vi "Mono Mirror.vi"(8 "error in (no error)":errorcluster, 11 "Mono In":refnum<class "Monochromator.lvclass">) -> (0 "error out":errorcluster, 2 "new Position":i32, 3 "Position":i32)   [LabVIEW 2020, in "Examples.lvlib"]
doc: "This example shows how to get and set the mirror position of the mono."
uses:
  Examples.lvlib
  Classes/Mono/Monochromator.lvclass
  0bd624ee-cc67-429d-86ba-aa8b37d700b1.vi
  01530acb-cdb4-4e7f-ad8c-3491b7af0b5d.vi
panel:
  in  "Stop":bool
  # "Connector Pane"
  # "Locals"
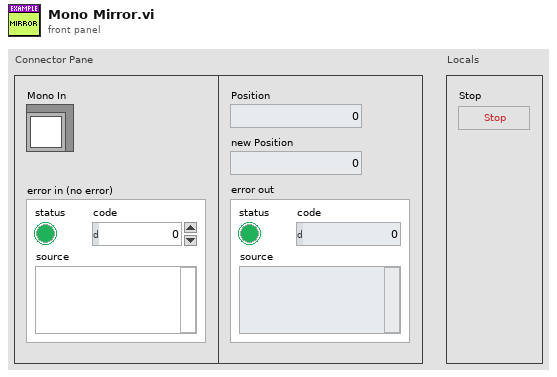
[diagram p1: front panel]
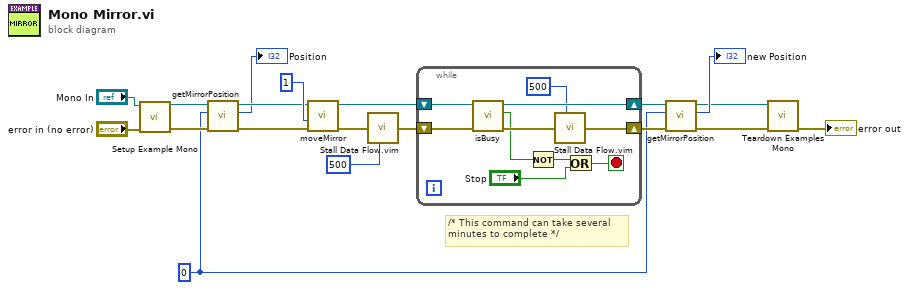
[diagram p0: block diagram]
diagram:
  w1 = 0 ("locationId")
  # "/* This command can take several \nminutes to complete */"
  n1 = call "Setup Example Mono.vi"("error in (no error)"="error in (no error)", "Mono In"="Mono In") -> ("error out"=w6:errorcluster, "Mono Out"=w4:refnum<class "Monochromator.lvclass">)  [unwired: 6 in, 2 out]
  n2 = call "getMirrorPosition.vi"("error in (no error)"=w6, "locationId"=w1, "Monochromator in"=w4) -> ("error out"=w5:errorcluster, "position"=→"Position":i32, "Monochromator out"=w3:refnum<class "Monochromator.lvclass">)  [unwired: 6 in]
  n3 = call "moveMirror.vi"("error in (no error)"=w5, "position"=1, "Monochromator in"=w3) -> ("error out"=w15:errorcluster, "Monochromator out"=w12:refnum<class "Monochromator.lvclass">)  [unwired: 5 in, 2 out]
  n4 = call "Stall Data Flow.vim"("value in"=w15, "milliseconds to wait"=u32 500) -> ("value out"=w14:errorcluster)  [unwired: 1 out]
  n5 = while {
    shift-right: [w25] -> w9
    shift-left: w14 -> [w27]
    shift-right: [w28] -> w10
    shift-left: w12 -> [w26]
    stop <- w22 stop-if-true
    n6 = call "isBusy.vi"("error in (no error)"=w27, "Monochromator in"=w26) -> ("error out"=w29:errorcluster, "mono is busy?"=w23:bool, "Monochromator out"=w28:refnum<class "Monochromator.lvclass">)  [unwired: 7 in]
    n7 = Not(x=w23) -> (.not. x?=w20:bool)
    n8 = call "Stall Data Flow.vim"("value in"=w29, "milliseconds to wait"=u32 500) -> ("value out"=w25:errorcluster)  [unwired: 1 out]
    n9 = Or(x=w20, y="Stop") -> (x .or. y?=w22:bool)
  }
  n10 = call "getMirrorPosition.vi"("error in (no error)"=w9, "locationId"=w1, "Monochromator in"=w10) -> ("error out"=w8:errorcluster, "position"=→"new Position":i32, "Monochromator out"=w7:refnum<class "Monochromator.lvclass">)  [unwired: 6 in]
  n11 = call "Teardown Examples Mono.vi"("error in (no error)"=w8, "Monochromator in"=w7) -> ("error out"=→"error out":errorcluster)  [unwired: 9 in]
